vi "Main.vi"() -> ()   [LabVIEW 2015]
doc: "This Continuous Measurement sample project is based on the Queued Message Handler template.\n\nThe Event Handling Loop generates messages based on user interface actions.\n\nThe Message Handling Loop processes messages generated by the Event Handling Loop, or by other messages. There are also Acquisition and Logging message handling loop subVIs, and a chart updating loop."
uses:
  Settings/Settings.ctl
  Acquisition/Hardware Configuration.ctl
  Acquisition/Signal Type.ctl
  Logging/Logging Configuration.ctl
  controls/UI Data.ctl
  controls/UI State.ctl
  support/Message Queue/Enqueue Message (Single).vi
  support/Message Queue/Enqueue Message (Array).vi
  <vilib>/Utility/error.llb/Error Cluster From Error Code.vi
  <vilib>/ErrorRing/Error Ring.xnode
  Acquisition/Acquisition.lvlib
  Logging/Logging.lvlib
  Settings/Settings.lvlib
  support/User Event - Stop/User Event - Stop.lvlib
  support/Message Queue/Message Queue.lvlib
  Settings/Settings Dialog.vi
panel:
  out "Data":waveform(dbl)[](graph)
  in  "Settings":bool
  in  "Start":bool
  in  "Stop":bool
  out "Status":string
  in  "Exit":bool
  # "Continuous Measurement Data Logger"
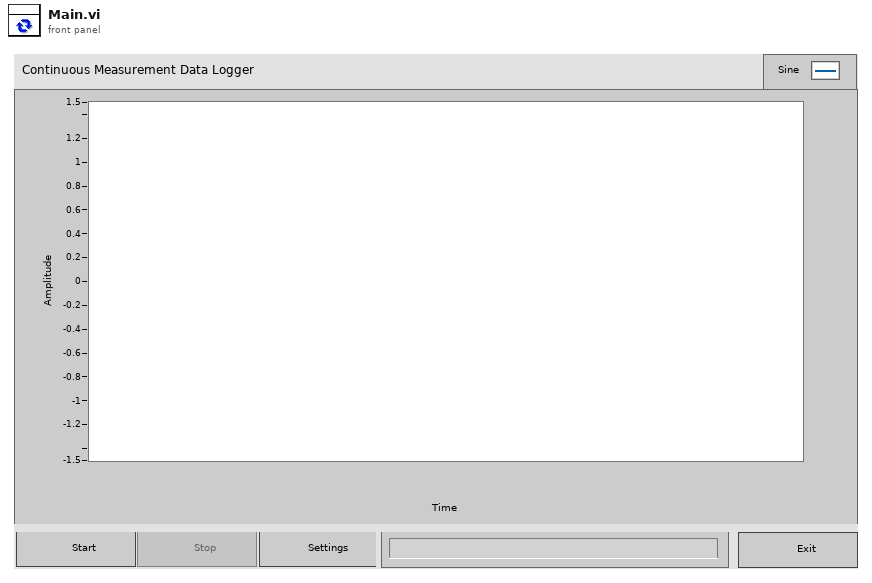
[diagram p1: front panel]
types:
  T1 = typedef "UI State.ctl" = enum16{"Idle", "Acquiring and Logging", "Waiting for Exit", "Waiting for Exit (Acq Stopped)", "Waiting for Exit (Log Stopped)", "Waiting for Stop", "Waiting for Stop (Acq Stopped)", "Waiting for Stop (Log Stopped)"}
  T2 = typedef "UI Data.ctl" = cluster{"Start Ref":refnum<vi>, "Stop Ref":refnum<vi>, "Settings Ref":refnum<vi>, "Exit Ref":refnum<vi>, "Status Ref":refnum<vi>, "Data Ref":refnum<vi>}
  T3 = typedef "Settings.lvlib/Settings.ctl" = cluster{"Hardware Configuration":T4, "Logging Configuration":T6}
  T4 = typedef "Acquisition.lvlib/Hardware Configuration.ctl" = cluster{"HW Refnum <Replace Me>":string, "Signal Type <Replace Me>":T5}
  T5 = typedef "Acquisition.lvlib/Signal Type.ctl" = enum16{"Sine Wave", "Square with Noise"}
  T6 = typedef "Logging.lvlib/Logging Configuration.ctl" = cluster{"Log File Base Path":path, "TDMS File Reference":refnum<k34>}
  T7 = typedef "Message Queue.lvlib/All Message Queues.ctl" = cluster{"UI":refnum<queue>, "Acquisition":refnum<queue>, "Logging":refnum<queue>}
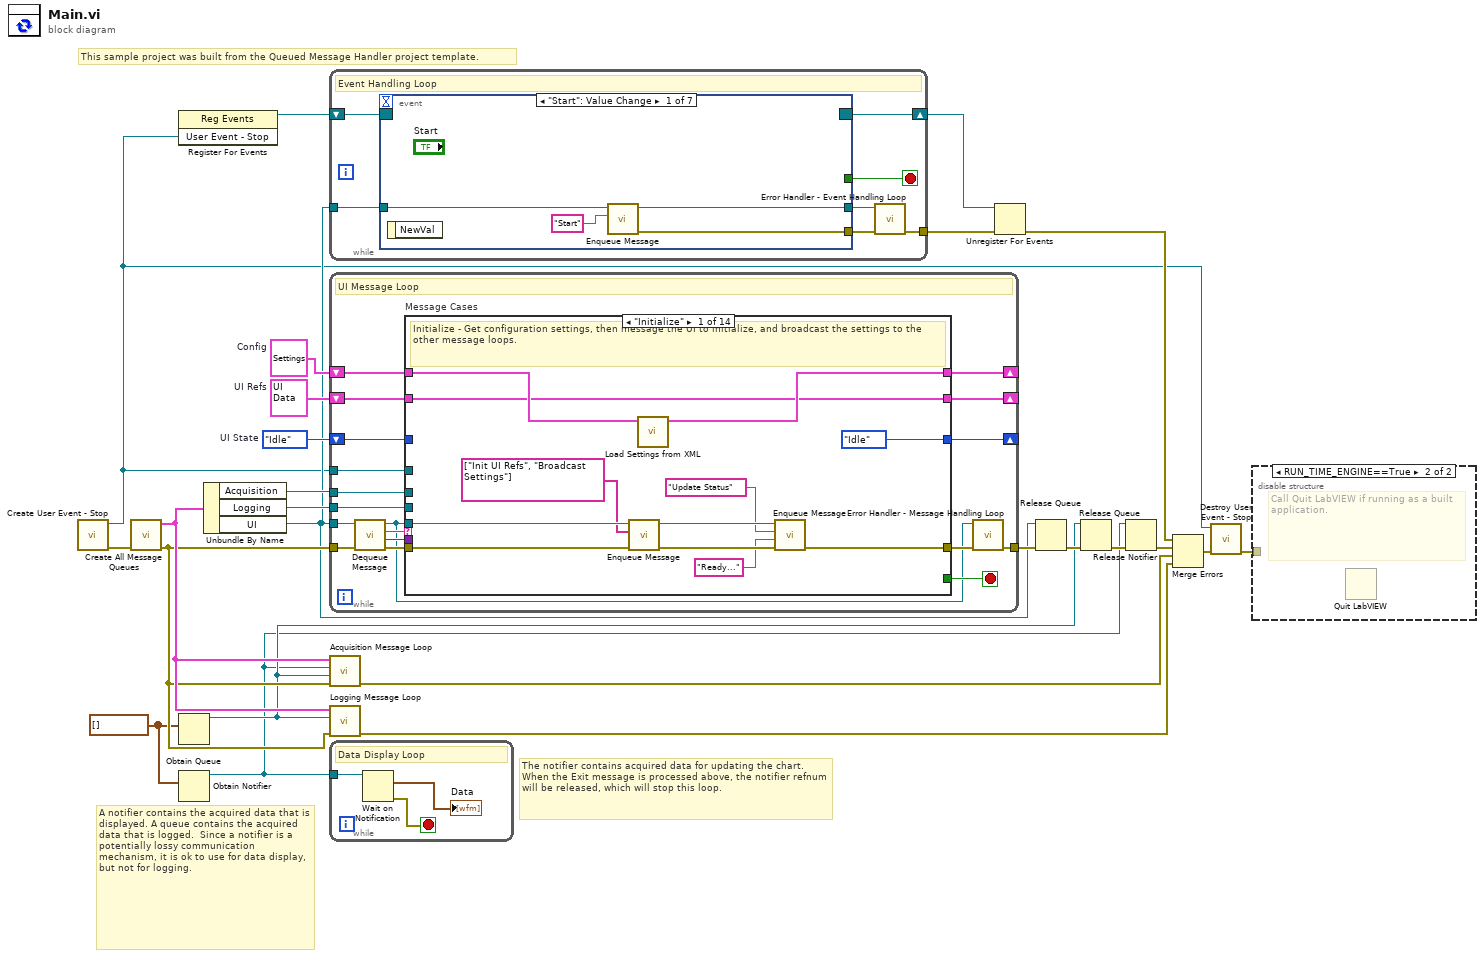
[diagram p0: block diagram]
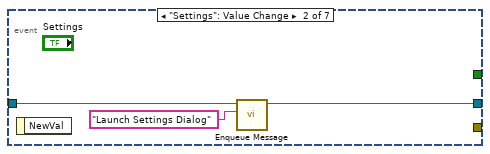
[diagram p3: hidden frame]
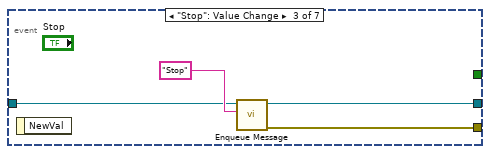
[diagram p4: hidden frame]
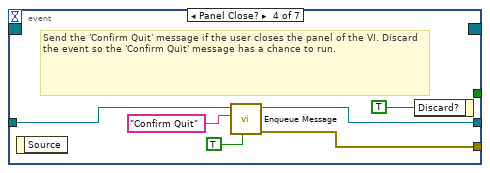
[diagram p5: hidden frame]
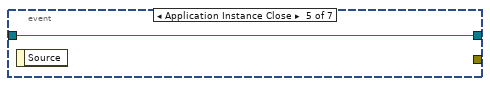
[diagram p6: hidden frame]
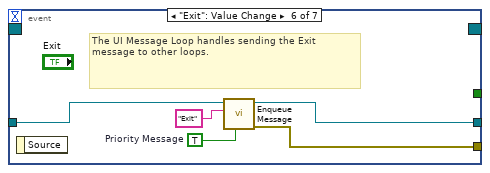
[diagram p7: hidden frame]
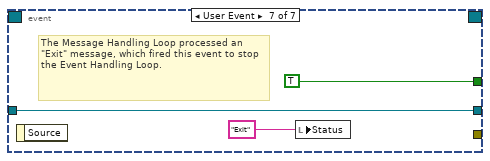
[diagram p8: hidden frame]
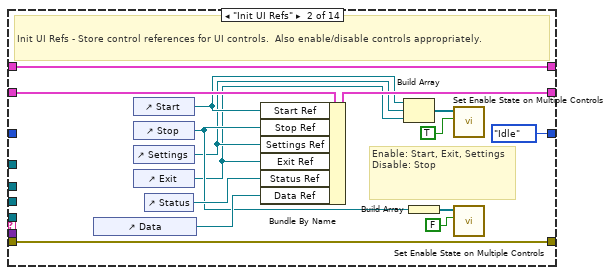
[diagram p9: hidden frame]
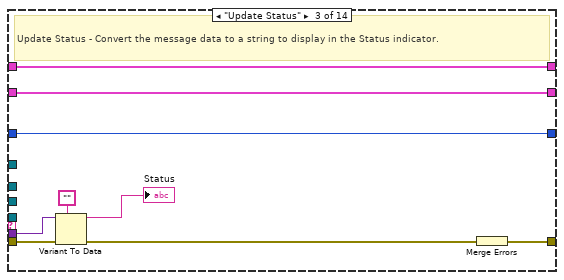
[diagram p10: hidden frame]
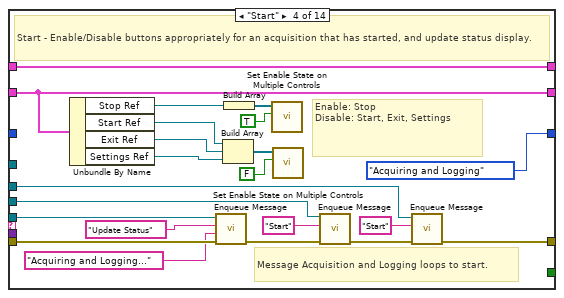
[diagram p11: hidden frame]
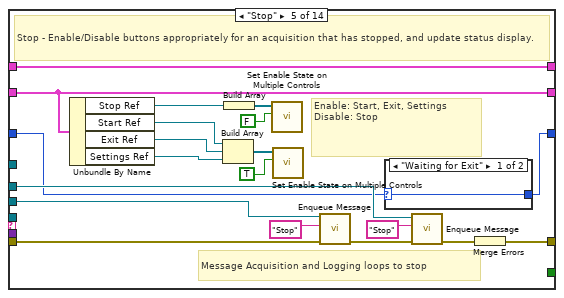
[diagram p12: hidden frame]
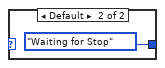
[diagram p13: hidden frame]
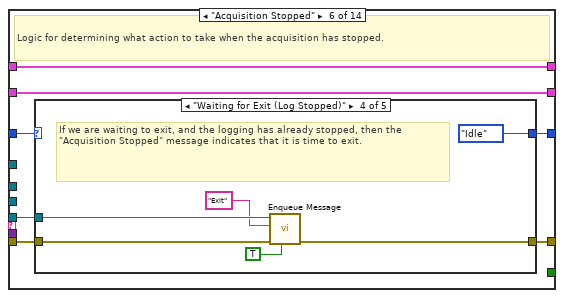
[diagram p14: hidden frame]
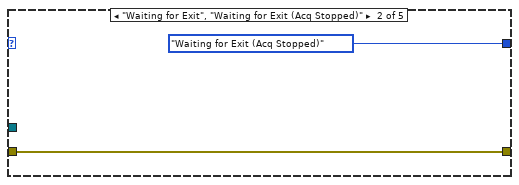
[diagram p16: hidden frame]
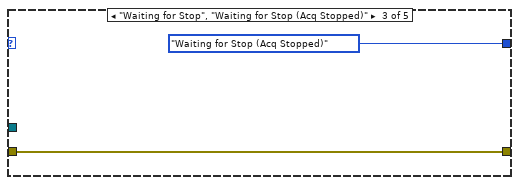
[diagram p17: hidden frame]
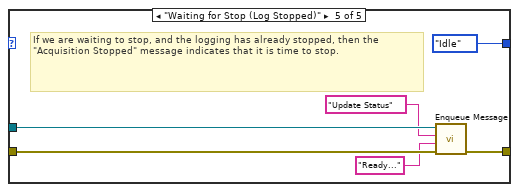
[diagram p18: hidden frame]
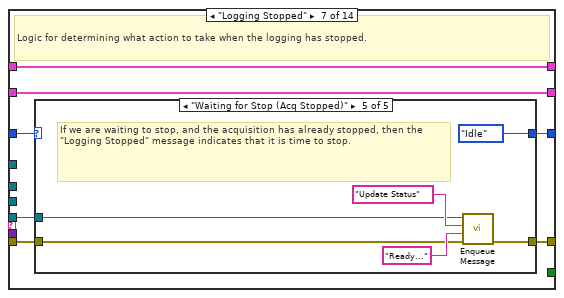
[diagram p19: hidden frame]
diagram:
  w12 = UI_State."Idle"  # UI State
  w3 = waveform(dbl)[] []
  w15 = T2 {"Start Ref"=refnum, "Stop Ref"=refnum, "Settings Ref"=refnum, "Exit Ref"=refnum, "Status Ref"=refnum, "Data Ref"=refnum}  # UI Refs
  w18 = T3 {"Hardware Configuration"={"HW Refnum <Replace Me>"="", "Signal Type <Replace Me>"=enum."Sine Wave"}, "Logging Configuration"={"Log File Base Path"=path "", "TDMS File Reference"=refnum}}  # Config
  # "This sample project was built from the Queued Message Handler project template."
  # "A notifier contains the acquired data that is displayed. A queue contains the acquired data that is logged.  Since a notifier is a potentially lossy communication mechanism, it is ok to use for data display, but not for logging."
  # "The notifier contains acquired data for updating the chart. When the Exit message is processed above, the notifier refnum will be released, which will stop this loop."
  n1 = call "Create User Event - Stop.vi"() -> ("error out"=w22:errorcluster, "User Event - Stop"=w1:refnum<user-event>)  [unwired: 10 in]
  n2 = call "Create All Message Queues.vi"("error in (no error)"=w22) -> ("error out"=w19:errorcluster, "Message Queues out"=w21:T7)  [unwired: 9 in]
  n3 = register-events(w1) -> (reference out=w2:refnum<event-registration>)  [unwired: 2 in, 1 out]
  n4 = Obtain Queue(element data type=w3) -> (queue out=w5:refnum<queue>)  [unwired: 4 in, 2 out]
  n5 = Obtain Notifier(notification data type=w3) -> (notifier out=w4:refnum<notifier>)  [unwired: 3 in, 2 out]
  n6 = Unbundle By Name(w21) -> ("Acquisition"=w14:refnum<queue>, "Logging"=w13:refnum<queue>, "UI"=w10:refnum<queue>)
  n7 = while {
    tunnel: w10 -> [w31]
    tunnel: [w28] -> w24
    shift-right: [w30] -> w16
    shift-left: w2 -> [w32]
    stop <- w29 stop-if-true
    # "Event Handling Loop"
    n8 = event shown="[0] \"Start\": Value Change" {
      selector: w32 -> [_ _ _ _ _ _ _]
      dyn-events: [_ _ _ _ _ _ _] -> w30
      timeout: _ -> [_ _ _ _ _ _ _]
      tunnel: [_ _ _ _ _ _ TRUE ("Discard?")] -> w29
      tunnel: w31 -> [w36 w38 w42 w47 w50 w52 w56]
      tunnel: [w34 _ w41 w45 _ w55 _] -> w27
      tunnel: [w33 w37 w40 w46 w50 w51 w56] -> w26
      event "Start": Value Change {
        n9 = event-data() -> ()  [unwired: 1 in, 1 out]
        n10 = call-poly "Enqueue Message.vi"("Message"="Start", "Message Queue"=w36) -> ("error out"=w34:errorcluster, "dup Message Queue"=w33:refnum<queue>)  [unwired: 8 in]
      }
      event "Settings": Value Change {
        n11 = event-data() -> ()  [unwired: 1 in, 1 out]
        n12 = call-poly "Enqueue Message.vi"("Message"="Launch Settings Dialog", "Message Queue"=w38) -> ("dup Message Queue"=w37:refnum<queue>)  [unwired: 8 in, 1 out]
      }
      event "Stop": Value Change {
        n13 = event-data() -> ()  [unwired: 1 in, 1 out]
        n14 = call-poly "Enqueue Message.vi"("Message"="Stop", "Message Queue"=w42) -> ("error out"=w41:errorcluster, "dup Message Queue"=w40:refnum<queue>)  [unwired: 8 in]
      }
      event Panel Close? {
        # "Send the 'Confirm Quit' message if the user closes the panel of the VI. Discard the event so the 'Confirm Quit' message has a chance to run."
        n15 = event-data() -> ()  [unwired: 1 in, 1 out]
        n16 = call-poly "Enqueue Message.vi"("Priority Message? (F)"=TRUE, "Message"="Confirm Quit", "Message Queue"=w47) -> ("error out"=w45:errorcluster, "dup Message Queue"=w46:refnum<queue>)  [unwired: 7 in]
        n17 = event-data("Discard?"=TRUE) -> ()  [unwired: 1 in, 1 out]
      }
      event Application Instance Close {
        n18 = event-data() -> ()  [unwired: 1 in, 1 out]
      }
      event "Exit": Value Change {
        w53 = TRUE  # Priority Message
        # "The UI Message Loop handles sending the Exit message to other loops."
        n19 = event-data() -> ()  [unwired: 1 in, 1 out]
        n20 = call-poly "Enqueue Message.vi"("Priority Message? (F)"=w53, "Message"="Exit", "Message Queue"=w52) -> ("error out"=w55:errorcluster, "dup Message Queue"=w51:refnum<queue>)  [unwired: 7 in]
      }
      event User Event {
        # "The Message Handling Loop processed an \"Exit\" message, which fired this event to stop the Event Handling Loop."
        n21 = event-data() -> ()  [unwired: 1 in, 1 out]
        n22 = local write "Status"("Exit" ("Exit String")) -> ()
      }
    }
    n23 = call "Error Handler - Event Handling Loop.vi"("error in (no error)"=w27, "Message Queue"=w26) -> ("dup error in"=w28:errorcluster)  [unwired: 8 in, 1 out]
  }
  n24 = while {
    tunnel: w10 -> [w70]
    tunnel: w1 -> [w75]
    shift-right: [w69] -> _
    shift-left: w18 -> [w68]
    shift-right: [w66] -> _
    shift-left: w15 -> [w67]
    tunnel: w14 -> [w65]
    tunnel: w13 -> [w64]
    shift-right: [w59] -> _
    shift-left: w12 -> [w60]
    tunnel: w19 -> [w74]
    tunnel: [w63] -> w25
    stop <- w76 stop-if-true
    # "UI Message Loop"
    n25 = call "Dequeue Message.vi"("error in (no error)"=w74, "Message Queue"=w70) -> ("error out"=w73:errorcluster, "Message Data"=w71:variant, "Message"=w72:string, "dup Message Queue"=w61:refnum<queue>)  [unwired: 6 in]
    n26 = case "Message Cases" shown="\"Initialize\"" w72 {
      selector: w72 -> [_ _ _ _ _ _ _ _ _ _ _ _ _ w292]
      tunnel: w61 -> [w80 _ _ w134 _ w159 w184 _ w224 _ w245 _ _ _]
      tunnel: w73 -> [w79 w103 w111 w133 w153 w160 w185 w212 w226 w233 w244 w273 w290 _]
      tunnel: [w84 w103 w112 w116 w154 w157 w182 w218 w219 w236 w243 w283 w289 w291] -> w62
      tunnel: [_ _ _ _ _ _ _ _ _ _ _ TRUE _ _] -> w76
      tunnel: w71 -> [_ _ w110 _ _ _ _ _ _ w237 _ w271 _ _]
      tunnel: w75 -> [_ _ _ _ _ _ _ _ _ _ _ w284 _ _]
      tunnel: [w87 w102 w106 w132 w152 w163 w188 w216 w223 w241 w248 w282 w288 w295] -> w69
      tunnel: w68 -> [w88 w102 w106 w132 w152 w163 w188 w216 w227 w241 w248 w282 w288 w295]
      tunnel: w67 -> [w81 w101 w105 w129 w151 w162 w187 w210 w221 w240 w247 w281 w287 w294]
      tunnel: [w81 w98 w105 w129 w151 w162 w187 w210 w221 w240 w247 w281 w287 w294] -> w66
      tunnel: w65 -> [_ _ _ w115 w138 _ _ w209 _ _ _ w280 _ _]
      tunnel: w64 -> [_ _ _ w118 w141 _ _ w208 _ _ _ w279 _ _]
      tunnel: w60 -> [_ _ w104 _ w135 w161 w186 w207 w220 w235 w246 _ w286 w293]
      tunnel: [UI_State."Idle" ("UI State") UI_State."Idle" ("UI State") w104 UI_State."Acquiring and Logging" ("UI State") w136 w158 w183 w207 w220 w235 w242 UI_State."Idle" ("UI State") w286 w293] -> w59
      frame "Initialize" {
        # "Initialize - Get configuration settings, then message the UI to initialize, and broadcast the settings to the other message loops."
        n27 = call-poly "Enqueue Message.vi"("error in (no error)"=w79, "Message Array"=string[] ["Init UI Refs", "Broadcast Settings"], "Message Queue"=w80) -> ("error out"=w86:errorcluster, "dup Message Queue"=w85:refnum<queue>)  [unwired: 7 in]
        n28 = call "Load Settings from XML.vi"("Settings in"=w88) -> ("Settings out"=w87:T3)  [unwired: 9 in, 1 out]
        n29 = call-poly "Enqueue Message.vi"("error in (no error)"=w86, "Message Data"="Ready..." ("Ready..."), "Message"="Update Status", "Message Queue"=w85) -> ("error out"=w84:errorcluster)  [unwired: 6 in, 1 out]
      }
      frame "Init UI Refs" {
        # "Enable: Start, Exit, Settings\nDisable: Stop"
        # "Init UI Refs - Store control references for UI controls.  Also enable/disable controls appropriately."
        n30 = control-ref of="Data"() -> (w99:refnum<vi>)
        n31 = control-ref of="Start"() -> (w92:refnum<vi>)
        n32 = control-ref of="Stop"() -> (w93:refnum<vi>)
        n33 = control-ref of="Settings"() -> (w91:refnum<vi>)
        n34 = control-ref of="Exit"() -> (w90:refnum<vi>)
        n35 = control-ref of="Status"() -> (w100:refnum<vi>)
        n36 = Bundle By Name(cluster=w101, "Start Ref"=w92, "Stop Ref"=w93, "Settings Ref"=w91, "Exit Ref"=w90, "Status Ref"=w100, "Data Ref"=w99) -> (w98:T2)
        n37 = Build Array(w92, w91, w90) -> (w96:refnum<vi>[])
        n38 = Build Array(w93) -> (w95:refnum<vi>[])
        n39 = call "Set Enable State on Multiple Controls.vi"("Enable?"=TRUE, "Controls"=w96) -> ()  [unwired: 10 in]
        n40 = call "Set Enable State on Multiple Controls.vi"("Enable?"=FALSE, "Controls"=w95) -> ()  [unwired: 10 in]
      }
      frame "Update Status" {
        # "Update Status - Convert the message data to a string to display in the Status indicator."
        n41 = Variant To Data(error in=w111, type="", Variant=w110) -> (data=→"Status":string, error out=w108:errorcluster)
        n42 = Merge Errors(w108) -> (w112:errorcluster)
      }
      frame "Start" {
        # "Message Acquisition and Logging loops to start."
        # "Enable: Stop\nDisable: Start, Exit, Settings"
        # "Start - Enable/Disable buttons appropriately for an acquisition that has started, and update status display."
        n43 = Unbundle By Name(w129) -> ("Stop Ref"=w124:refnum<vi>, "Start Ref"=w123:refnum<vi>, "Exit Ref"=w122:refnum<vi>, "Settings Ref"=w121:refnum<vi>)
        n44 = call-poly "Enqueue Message.vi"("error in (no error)"=w133, "Message Data"="Acquiring and Logging..." ("Acquiring and Logging..."), "Message"="Update Status", "Message Queue"=w134) -> ("error out"=w120:errorcluster)  [unwired: 6 in, 1 out]
        n45 = Build Array(w123, w122, w121) -> (w127:refnum<vi>[])
        n46 = Build Array(w124) -> (w126:refnum<vi>[])
        n47 = call "Set Enable State on Multiple Controls.vi"("Enable?"=TRUE, "Controls"=w126) -> ()  [unwired: 10 in]
        n48 = call "Set Enable State on Multiple Controls.vi"("Enable?"=FALSE, "Controls"=w127) -> ()  [unwired: 10 in]
        n49 = call-poly "Enqueue Message.vi"("error in (no error)"=w120, "Message"="Start", "Message Queue"=w118) -> ("error out"=w117:errorcluster)  [unwired: 7 in, 1 out]
        n50 = call-poly "Enqueue Message.vi"("error in (no error)"=w117, "Message"="Start", "Message Queue"=w115) -> ("error out"=w116:errorcluster)  [unwired: 7 in, 1 out]
      }
      frame "Stop" {
        # "Message Acquisition and Logging loops to stop"
        # "Enable: Start, Exit, Settings\nDisable: Stop"
        # "Stop - Enable/Disable buttons appropriately for an acquisition that has stopped, and update status display."
        n51 = Unbundle By Name(w151) -> ("Stop Ref"=w146:refnum<vi>, "Start Ref"=w145:refnum<vi>, "Exit Ref"=w144:refnum<vi>, "Settings Ref"=w143:refnum<vi>)
        n52 = Build Array(w145, w144, w143) -> (w149:refnum<vi>[])
        n53 = Build Array(w146) -> (w148:refnum<vi>[])
        n54 = call "Set Enable State on Multiple Controls.vi"("Enable?"=FALSE, "Controls"=w148) -> ()  [unwired: 10 in]
        n55 = call "Set Enable State on Multiple Controls.vi"("Enable?"=TRUE, "Controls"=w149) -> ()  [unwired: 10 in]
        n56 = call-poly "Enqueue Message.vi"("error in (no error)"=w153, "Message"="Stop", "Message Queue"=w141) -> ("error out"=w140:errorcluster)  [unwired: 7 in, 1 out]
        n57 = case shown="\"Waiting for Exit\"" w135 {
          selector: w135 -> [w155 _]
          tunnel: [w155 UI_State."Waiting for Stop" ("UI State")] -> w136
          frame "Waiting for Exit" {
          }
          frame Default {
          }
        }
        n58 = call-poly "Enqueue Message.vi"("error in (no error)"=w140, "Message"="Stop", "Message Queue"=w138) -> ("error out"=w139:errorcluster)  [unwired: 7 in, 1 out]
        n59 = Merge Errors(w139) -> (w154:errorcluster)
      }
      frame "Acquisition Stopped" {
        # "Logic for determining what action to take when the acquisition has stopped."
        n60 = case shown="\"Waiting for Exit (Log Stopped)\"" w161 {
          selector: w161 -> [w165 _ _ _ _]
          tunnel: w160 -> [w164 w167 w169 w175 w181]
          tunnel: w159 -> [_ _ _ w173 w178]
          tunnel: [w165 UI_State."Waiting for Exit (Acq Stopped)" ("UI State") UI_State."Waiting for Stop (Acq Stopped)" ("UI State") UI_State."Idle" ("UI State") UI_State."Idle" ("UI State")] -> w158
          tunnel: [w164 w167 w169 w174 w179] -> w157
          frame Default {
          }
          frame "Waiting for Exit", "Waiting for Exit (Acq Stopped)" {
          }
          frame "Waiting for Stop", "Waiting for Stop (Acq Stopped)" {
          }
          frame "Waiting for Exit (Log Stopped)" {
            # "If we are waiting to exit, and the logging has already stopped, then the \"Acquisition Stopped\" message indicates that it is time to exit."
            n61 = call-poly "Enqueue Message.vi"("Priority Message? (F)"=TRUE, "error in (no error)"=w175, "Message"="Exit", "Message Queue"=w173) -> ("error out"=w174:errorcluster)  [unwired: 6 in, 1 out]
          }
          frame "Waiting for Stop (Log Stopped)" {
            # "If we are waiting to stop, and the logging has already stopped, then the \"Acquisition Stopped\" message indicates that it is time to stop."
            n62 = call-poly "Enqueue Message.vi"("error in (no error)"=w181, "Message Data"="Ready..." ("Ready..."), "Message"="Update Status", "Message Queue"=w178) -> ("error out"=w179:errorcluster)  [unwired: 6 in, 1 out]
          }
        }
      }
      frame "Logging Stopped" {
        # "Logic for determining what action to take when the logging has stopped."
        n63 = case shown="\"Waiting for Stop (Acq Stopped)\"" w186 {
          selector: w186 -> [w190 _ _ _ _]
          tunnel: w185 -> [w189 w192 w194 w200 w203]
          tunnel: w184 -> [_ _ _ w198 w202]
          tunnel: [w190 UI_State."Waiting for Exit (Log Stopped)" ("UI State") UI_State."Waiting for Stop (Log Stopped)" ("UI State") UI_State."Idle" ("UI State") UI_State."Idle" ("UI State")] -> w183
          tunnel: [w189 w192 w194 w199 w201] -> w182
          frame Default {
          }
          frame "Waiting for Exit", "Waiting for Exit (Log Stopped)" {
          }
          frame "Waiting for Stop", "Waiting for Stop (Log Stopped)" {
          }
          frame "Waiting for Exit (Acq Stopped)" {
            # "If we are waiting to exit, and the acquisition has already stopped, then the \"Logging Stopped\" message indicates that it is time to exit."
            n64 = call-poly "Enqueue Message.vi"("Priority Message? (F)"=TRUE, "error in (no error)"=w200, "Message"="Exit", "Message Queue"=w198) -> ("error out"=w199:errorcluster)  [unwired: 6 in, 1 out]
          }
          frame "Waiting for Stop (Acq Stopped)" {
            # "If we are waiting to stop, and the acquisition has already stopped, then the \"Logging Stopped\" message indicates that it is time to stop."
            n65 = call-poly "Enqueue Message.vi"("error in (no error)"=w203, "Message Data"="Ready..." ("Ready..."), "Message"="Update Status", "Message Queue"=w202) -> ("error out"=w201:errorcluster)  [unwired: 6 in, 1 out]
          }
        }
      }
      frame "Broadcast settings" {
        w211 = "Update Settings" ("Message")
        # "Broadcast settings - Send the 'Update Settings' message to the Logging and Acquisition message loops."
        n66 = Unbundle By Name(w216) -> ("Hardware Configuration"=w215:T4, "Logging Configuration"=w214:T6)
        n67 = call-poly "Enqueue Message.vi"("Message Data"=w215, "Message"=w211, "Message Queue"=w209) -> ("error out"=w217:errorcluster)  [unwired: 7 in, 1 out]
        n68 = call-poly "Enqueue Message.vi"("error in (no error)"=w217, "Message Data"=w214, "Message"=w211, "Message Queue"=w208) -> ("error out"=w213:errorcluster)  [unwired: 6 in, 1 out]
        n69 = Merge Errors(w213, w212) -> (w218:errorcluster)
      }
      frame "Launch Settings Dialog" {
        # "Launch Settings Dialog - Launch the Settings Dialog when the user clicks the 'Settings' button."
        n70 = call-by-ref "?"("error in (no error)"=w226, "Settings in"=w227) -> ("error out"=w222:errorcluster, "Cancelled?"=w225:bool, "Settings out"=w223:T3)  [unwired: 8 in, 3 out]
        n71 = case shown="False" w225 {
          tunnel: w224 -> [w231 _]
          tunnel: w222 -> [w230 w232]
          tunnel: [w229 w232] -> w219
          frame False {
            n72 = call-poly "Enqueue Message.vi"("error in (no error)"=w230, "Message"="Broadcast Settings", "Message Queue"=w231) -> ("error out"=w229:errorcluster)  [unwired: 7 in, 1 out]
          }
          frame True {
          }
        }
      }
      frame "Error" {
        # "Error - Display an error dialog. This message is sent by the \"Error Handler\" VIs at the end of other loops in this application."
        n73 = Variant To Data(error in=w233, type=errorcluster {"status"=FALSE, "code"=0, "source"=""} ("error constant"), Variant=w237) -> (data=w234:errorcluster, error out=w238:errorcluster)
        n74 = call <vilib>:"Simple Error Handler.vi"("error in (no error)"=w234) -> ()  [unwired: 4 in, 5 out]
        n75 = Merge Errors(w238) -> (w236:errorcluster)
      }
      frame "Confirm Quit" {
        # "Confirm Quit - Message that can confirm whether or not the user wants to exit the application."
        n76 = case shown="\"Acquiring and Logging\"" w246 {
          tunnel: w245 -> [w254 w258]
          tunnel: w244 -> [w253 w257]
          tunnel: [w252 w256] -> w243
          tunnel: [UI_State."Idle" ("UI State") w255] -> w242
          frame Default {
            # "If 'Confirm Quit' comes in while the system is idle, there is no need for a confirmation message."
            n77 = call-poly "Enqueue Message.vi"("Priority Message? (F)"=TRUE, "error in (no error)"=w253, "Message"="Exit", "Message Queue"=w254) -> ("error out"=w252:errorcluster)  [unwired: 6 in, 1 out]
          }
          frame "Acquiring and Logging" {
            n78 = Two Button Dialog(message="Are you sure you want to quit while the acquisition is running?" ("Confirm Quit Message"), 1:"No" ("No"), 2:"Yes" ("Yes")) -> (T button?=w259:bool)
            n79 = case shown="True" w259 {
              tunnel: w258 -> [_ w268]
              tunnel: w257 -> [w264 w269]
              tunnel: [w264 w267] -> w256
              tunnel: [UI_State."Acquiring and Logging" ("UI State") UI_State."Waiting for Exit" ("UI State")] -> w255
              frame False {
                # "User did not want to quit."
              }
              frame True {
                n80 = call-poly "Enqueue Message.vi"("error in (no error)"=w269, "Message"="Stop", "Message Queue"=w268) -> ("error out"=w267:errorcluster)  [unwired: 7 in, 1 out]
              }
            }
          }
        }
      }
      frame "Exit" {
        w275 = TRUE ("Priority Message? (F)")
        w276 = "Exit" ("Message")
        # "Popup an error dialog if 'Exit' was called as a result of an error."
        # "Stop the VI"
        # "Exit - Send Exit messages to the Acquisition and Logging loops, and fire the user event to stop the Event Handling Loop."
        n81 = Variant To Data(type=errorcluster {"status"=FALSE, "code"=0, "source"=""} ("error constant"), Variant=w271) -> (data=w270:errorcluster)  [unwired: 1 in, 1 out]
        n82 = call <vilib>:"Simple Error Handler.vi"("error in (no error)"=w270) -> ()  [unwired: 4 in, 5 out]
        n83 = call-poly "Enqueue Message.vi"("Priority Message? (F)"=w275, "error in (no error)"=w273, "Message"=w276, "Message Queue"=w280) -> ("error out"=w277:errorcluster)  [unwired: 6 in, 1 out]
        n84 = call-poly "Enqueue Message.vi"("Priority Message? (F)"=w275, "error in (no error)"=w277, "Message"=w276, "Message Queue"=w279) -> ("error out"=w274:errorcluster)  [unwired: 6 in, 1 out]
        n85 = call "Fire User Event - Stop.vi"("error in (no error)"=w274, "User Event - Stop"=w284) -> ("error out"=w283:errorcluster)  [unwired: 9 in]
      }
      frame "---Copy This Frame---" {
        # "Duplicate this frame when creating new messages.  Change this comment in the duplicated frame to describe this message."
        n86 = Merge Errors(w290) -> (w289:errorcluster)
      }
      frame Default {
        # "'Default' case only runs if there is a message that isn't defined in any of the other cases.  Output a programming error."
        n87 = xnode "Error Ring"("parameter 0"=w292) -> ("error out"=w291:errorcluster)
      }
    }
    n88 = call "Error Handler - Message Handling Loop.vi"("error in (no error)"=w62, "Message Queue"=w61) -> ("dup error in"=w63:errorcluster)  [unwired: 8 in, 1 out]
  }
  n89 = call "Acquisition Message Loop.vi"("error in (no error)"=w19, "Data Queue"=w5, "Data Notifier"=w4, "Message Queues"=w21) -> ("error out"=w23:errorcluster)  [unwired: 7 in]
  n90 = call "Logging Message Loop.vi"("error in (no error)"=w19, "Data Queue"=w5, "Message Queues"=w21) -> ("error out"=w20:errorcluster)  [unwired: 8 in]
  n91 = while "Data Display Loop" {
    tunnel: w4 -> [w305]
    stop <- w303 stop-if-true
    # "Data Display Loop"
    n92 = Wait on Notification(notifier=w305) -> (notification=→"Data":waveform(dbl)[], error out=w303:errorcluster)  [unwired: 3 in, 2 out]
  }
  n93 = Unregister For Events(event registration refnum=w16, error in=w24) -> (error out=w17:errorcluster)
  n94 = Release Queue(queue=w10, error in (no error)=w25) -> (error out=w8:errorcluster)  [unwired: 1 in, 2 out]
  n95 = Release Queue(queue=w5, error in (no error)=w8) -> (error out=w7:errorcluster)  [unwired: 1 in, 2 out]
  n96 = Release Notifier(notifier=w4, error in (no error)=w7) -> (error out=w6:errorcluster)  [unwired: 1 in, 2 out]
  n97 = Merge Errors(w17, w6, w23, w20) -> (w11:errorcluster)
  n98 = call "Destroy User Event - Stop.vi"("error in (no error)"=w11, "User Event - Stop"=w1) -> ("error out"=w9:errorcluster)  [unwired: 9 in]
  n99 = disable-structure shown="RUN_TIME_ENGINE==True" {
    disable-tunnel: w9 -> [_ _]
    frame condition #0 (active) {
    }
    frame condition #1 {
      # "Call Quit LabVIEW if running as a built application."
      n100 = Quit LabVIEW() -> ()  [unwired: 1 in]
    }
  }
